vi "Avail List.set.vi"(8 "error in (no error)":errorcluster, 10 "detail map":T1, 11 "selection_dropdown in":refnum<class "selection_dropdown.lvclass">) -> (0 "error out":errorcluster, 3 "selection_dropdown out":refnum<class "selection_dropdown.lvclass">)   [LabVIEW 2024, in "selection_dropdown.lvclass"]
uses:
  selection_dropdown.lvclass
  comic_manager/manager_daemon/type_defs/sub-map--map.ctl
  comic_manager/manager_daemon/type_defs/SubData--cluster.ctl
  selection_dropdown.lvclass/selection_dropdown.ctl
  comic_manager/manager_daemon/manager_daemon.lvclass
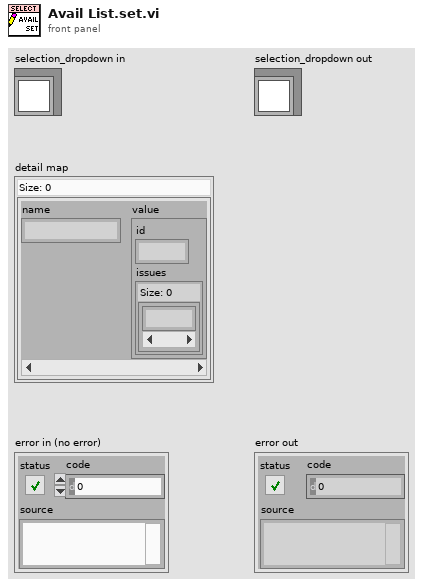
[diagram p1: front panel]
types:
  T1 = typedef "manager_daemon.lvclass/sub-map--map.ctl" = map{string, T2}
  T2 = typedef "manager_daemon.lvclass/SubData--cluster.ctl" = cluster{"id":i32, "issues":set{i32}}
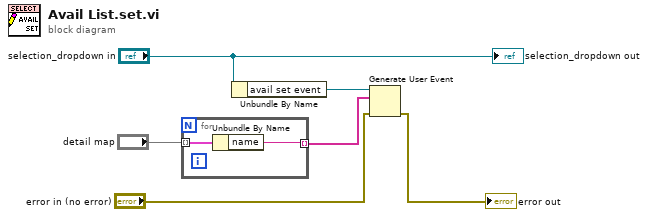
[diagram p0: block diagram]
diagram:
  n1 = for {
    tunnel: "detail map" -> [w8] mode=indexing
    tunnel: [w7] -> w1 mode=indexing
    n2 = Unbundle By Name(w8) -> ("name"=w7:string)
  }
  n3 = Unbundle By Name("selection_dropdown in") -> ("avail set event"=w5:refnum<user-event>)
  n4 = Generate User Event(user event=w5, event data cluster=w1, error in="error in (no error)") -> (error out=→"error out":errorcluster)  [unwired: 1 in, 1 out]
  "selection_dropdown out" <- "selection_dropdown in"
